vi "processEvt.vi"(8 "error in (no error)":errorcluster, 10 "tcpPacket":T1, 11 "tcpServerCmd in":refnum<class "TcpServerCmd.lvclass">) -> (0 "error out":errorcluster, 3 "tcpServerCmd out":refnum<class "TcpServerCmd.lvclass">)   [LabVIEW 2018, in "TcpServerCmd.lvclass"]
doc: "Process the incoming event. If event is already registered, it will be sent to LabVIEW Component as an user event."
uses:
  TcpServerCmd.lvclass
  home/pcortes/github/ts_labview_tcp_json/src/TcpServerBase/TcpServerBase.lvclass
  TcpServerBase/typedef/tcpPacketTypeDef.ctl
  TcpServerCmd.lvclass/TcpServerCmd.ctl
  TcpServerBase/TcpServerBase.lvclass
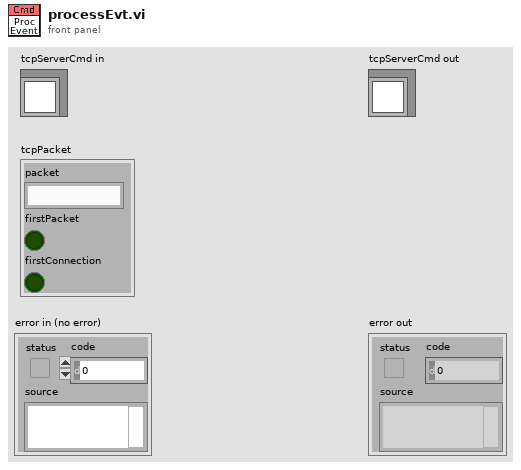
[diagram p1: front panel]
types:
  T1 = typedef "TcpServerBase.lvclass/tcpPacketTypeDef.ctl" = cluster{"packet":string, "firstPacket":bool, "firstConnection":bool}
  T2 = typedef "TcpServerCmd.lvclass/userEventTypeDef.ctl" = cluster{"CmdRead":refnum<user-event>, "CmdWrite":refnum<user-event>, "EvtRead":refnum<user-event>, "EvtWrite":refnum<user-event>, "GenRead":refnum<user-event>, "GenWrite":refnum<user-event>}
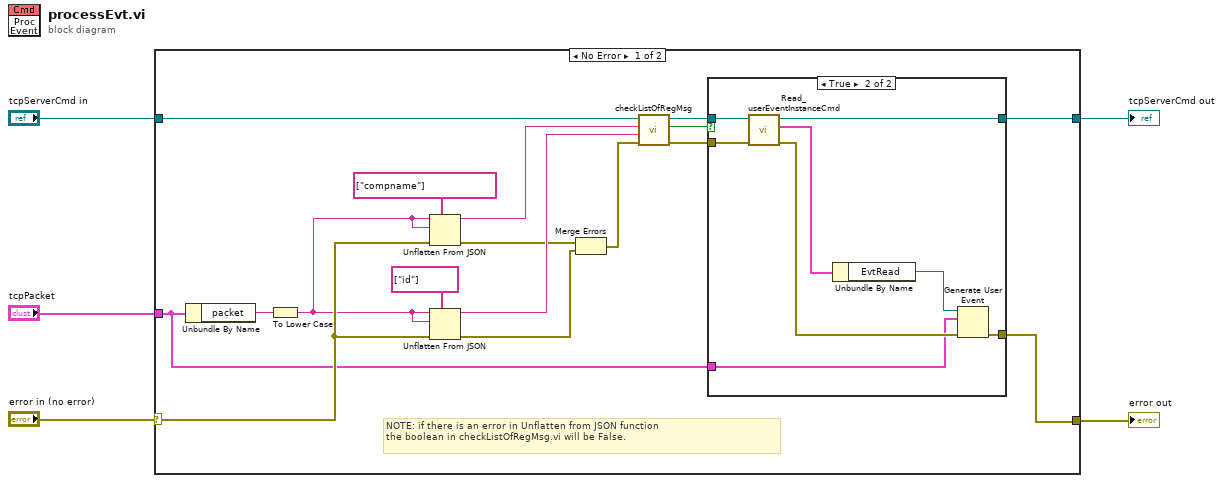
[diagram p0: block diagram]
diagram:
  n1 = case shown="No Error" "error in (no error)" {
    selector: "error in (no error)" -> [w18 w34]
    tunnel: [w7 w34] -> w4
    tunnel: [w14 w33] -> w2
    tunnel: "tcpServerCmd in" -> [w21 w33]
    tunnel: "tcpPacket" -> [w11 _]
    frame No Error {
      # "NOTE: if there is an error in Unflatten from JSON function\nthe boolean in checkListOfRegMsg.vi will be False."
      n2 = Unbundle By Name(w11) -> ("packet"=w19:string)
      n3 = To Lower Case(string=w19) -> (all lower case string=w6:string)
      n4 = Unflatten From JSON(path=string[] ["compname"] ("tcp packet"), JSON string=w6, type and defaults=w6, error in (no error)=w18) -> (value=w17:string, error out=w10:errorcluster)  [unwired: 3 in]
      n5 = Unflatten From JSON(path=string[] ["id"] ("tcp packet"), JSON string=w6, type and defaults=w6, error in (no error)=w18) -> (value=w16:string, error out=w8:errorcluster)  [unwired: 3 in]
      n6 = Merge Errors(w10, w8) -> (w9:errorcluster)
      n7 = call "checkListOfRegMsg.vi"("error in (no error)"=w9, "id"=w16, "compName"=w17, "tcpServerBase in"=w21) -> ("error out"=w13:errorcluster, "msgRegistered?"=w12:bool, "tcpServerBase out"=w15:refnum<class "TcpServerCmd.lvclass">)  [unwired: 5 in]
      n8 = case shown="True" w12 {
        tunnel: w15 -> [w24 w29]
        tunnel: [w24 w28] -> w14
        tunnel: w13 -> [w23 w27]
        tunnel: w11 -> [_ w26]
        tunnel: [w23 w25] -> w7
        frame False {
        }
        frame True {
          n9 = call "Read_userEventInstanceCmd.vi"("error in (no error)"=w27, "TcpServerCmd in"=w29) -> ("error out"=w30:errorcluster, "userEventInstance"=w31:T2, "TcpServerCmd out"=w28:refnum<class "TcpServerCmd.lvclass">)  [unwired: 7 in]
          n10 = Unbundle By Name(w31) -> ("EvtRead"=w32:refnum<user-event>)
          n11 = Generate User Event(user event=w32, event data cluster=w26, error in=w30) -> (error out=w25:errorcluster)  [unwired: 1 in, 1 out]
        }
      }
    }
    frame Error {
    }
  }
  "error out" <- w4
  "tcpServerCmd out" <- w2
